vi "Serial Receive.vi"(6 "ready for output":bool, 7 "clock sampling edge":enum16{"rising", "falling"}(ring)=enum."falling", 8 "transfer length":u8, 9 "force stop (F)":bool, 10 "start transfer":bool, 11 "signals in":cluster{"clock":bool, "data":bool}) -> (1 "output valid":bool, 3 "sample out":u32)   [LabVIEW 2013, in "I2S-TDM.lvlib"]
uses:
  I2S-TDM.lvlib
  Controls/serial receive states.ctl
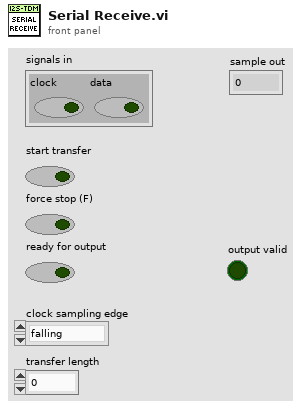
[diagram p1: front panel]
types:
  T1 = typedef "I2S-TDM.lvlib/serial receive states.ctl" = enum16{"idle", "transfer"}
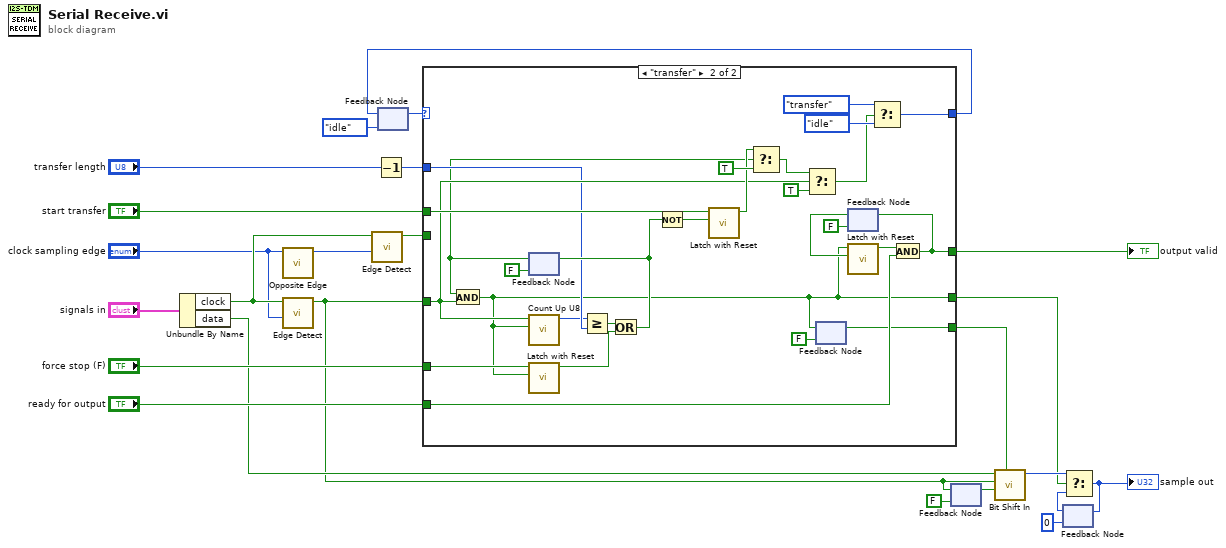
[diagram p0: block diagram]
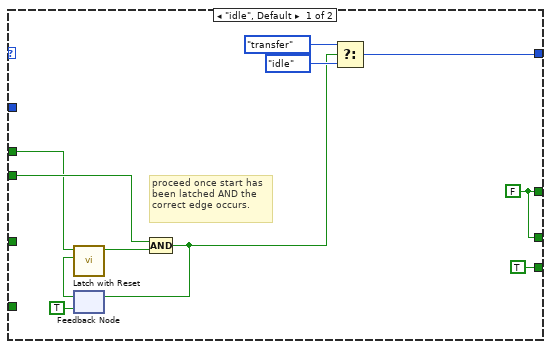
[diagram p2: hidden frame]
diagram:
  n1 = Unbundle By Name("signals in") -> ("clock"=w9:bool, "data"=w11:bool)
  n2 = call "Opposite Edge.vi"("edge in"="clock sampling edge") -> ("opposite edge out"=w7:enum16{"rising", "falling"})  [unwired: 10 in]
  n3 = call "Edge Detect.vi"("edge (rising)"="clock sampling edge", "signal in"=w9) -> ("edge detected?"=w5:bool)  [unwired: 9 in]
  n4 = call "Edge Detect.vi"("edge (rising)"=w7, "signal in"=w9) -> ("edge detected?"=w6:bool)  [unwired: 9 in]
  n5 = Decrement(x="transfer length") -> (x-1=w1:u8)
  n6 = feedback #1(serial_receive_states."idle" ("receive state")) -> (w13:T1)
  n7 = case shown="\"transfer\"" w13 {
    tunnel: [w35 w60] -> w23
    tunnel: w5 -> [_ w40]
    tunnel: "start transfer" -> [w29 w58]
    tunnel: [w31 w51] -> w16
    tunnel: "ready for output" -> [_ w52]
    tunnel: [TRUE ("rising edge?") w49] -> w10
    tunnel: w1 -> [_ w39]
    tunnel: [w31 w36] -> w15
    tunnel: "force stop (F)" -> [_ w57]
    tunnel: w6 -> [w30 _]
    frame "idle", Default {
      w31 = FALSE
      # "proceed once start has been latched AND the correct edge occurs."
      n8 = feedback #2(TRUE) -> (w26:bool)
      n9 = call "Latch with Reset.vi"("reset"=w26, "signal"=w29) -> ("latched signal"=w32:bool)  [unwired: 9 in]
      n10 = Compound Arithmetic op=AND(w30, w32) -> (w27:bool)
      n11 = feedback-in #2(w27) -> ()
      n12 = Select(t=serial_receive_states."transfer" ("receive state"), s=w27, f=serial_receive_states."idle" ("receive state")) -> (s? t:f=w35:T1)
    }
    frame "transfer" {
      n13 = feedback #3(FALSE) -> (w37:bool)
      n14 = And(x=w37, y=w40) -> (x .and. y?=w36:bool)
      n15 = call "Count Up U8.vi"("reset (F)"=w36, "increment"=w40) -> ("count"=w38:u8)  [unwired: 9 in]
      n16 = call "Latch with Reset.vi"("reset"=w36, "signal"=w57) -> ("latched signal"=w53:bool)  [unwired: 9 in]
      n17 = Greater Or Equal?(x=w38, y=w39) -> (x >= y?=w56:bool)
      n18 = Or(x=w56, y=w53) -> (x .or. y?=w41:bool)
      n19 = feedback-in #3(w41) -> ()
      n20 = Not(x=w41) -> (.not. x?=w45:bool)
      n21 = call "Latch with Reset.vi"("reset"=w45, "signal"=w58) -> ("latched signal"=w43:bool)  [unwired: 9 in]
      n22 = Select(t=w43, s=w37, f=TRUE) -> (s? t:f=w42:bool)
      n23 = Select(t=w42, s=w40, f=TRUE) -> (s? t:f=w47:bool)
      n24 = feedback-in #4(w36) -> ()
      n25 = feedback #4(FALSE ("rising edge?")) -> (w49:bool)
      n26 = feedback #5(FALSE) -> (w50:bool)
      n27 = call "Latch with Reset.vi"("reset"=w50, "signal"=w36) -> ("latched signal"=w54:bool)  [unwired: 9 in]
      n28 = Select(t=serial_receive_states."transfer" ("receive state"), s=w47, f=serial_receive_states."idle" ("receive state")) -> (s? t:f=w60:T1)
      n29 = And(x=w54, y=w52) -> (x .and. y?=w51:bool)
      n30 = feedback-in #5(w51) -> ()
    }
  }
  "output valid" <- w16
  n31 = feedback-in #1(w23) -> ()
  n32 = feedback-in #6(w5) -> ()
  n33 = feedback #6(FALSE ("edge detected?")) -> (w4:bool)
  n34 = call "Bit Shift In.vi"("reset"=w10, "shift index"=w4, "sample bit"=w5, "data bit in"=w11) -> ("sample"=w20:u32)  [unwired: 7 in]
  n35 = feedback #7(u32 0 ("sample")) -> (w19:u32)
  n36 = Select(t=w20, s=w15, f=w19) -> (s? t:f=w17:u32)
  "sample out" <- w17
  n37 = feedback-in #7(w17) -> ()
